vi "Stop Measurement.vi"(8 "error in":errorcluster, 10 "call id":T1, 11 "gRPCid in":T1) -> (0 "error out":errorcluster, 3 "gRPCid out":T1)   [LabVIEW 2021, in "MeasurementServerTests.lvlib" / "Measurement Service Tests.lvlib" / "Continuous Counting Client.lvlib"]
doc: "Stop the measurement."
uses:
  Continuous Counting Client.lvlib
  <vilib>/gRPC/LabVIEW gRPC Library/Shared/grpcId.ctl
  <vilib>/gRPC/LabVIEW gRPC Library/grpc-lvsupport-release.lvlib
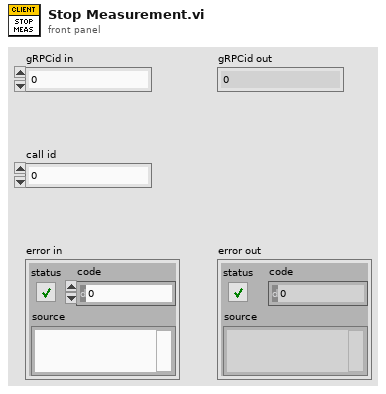
[diagram p1: front panel]
types:
  T1 = typedef "grpc-lvsupport-release.lvlib/grpcId.ctl" = u64
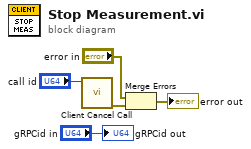
[diagram p0: block diagram]
diagram:
  n1 = call <vilib>:"Client Cancel Call.vi"("Call ID in"="call id") -> ("error out"=w2:errorcluster)  [unwired: 8 in, 2 out]
  n2 = Merge Errors("error in", w2) -> (→"error out":errorcluster)
  "gRPCid out" <- "gRPCid in"
